vi "Square_Difference_Filter(SDisp)-2.vi"(5 "X,Y":dbl[][](array[numeric]), 6 "[IN] Dot matrix with \nstatuses for potentially \nmoving dots":i16[][](array[numeric]), 7 "Areas":dbl[][](array[numeric]), 8 "error IN":errorcluster, 9 "[IN] Possibly\nMoving (X,Y)":dbl[][](array[numeric]), 10 "% DIfference between \nParticle Squares":dbl, 11 "(X,Y,dX,dY) In":dbl[][](array[numeric])) -> (0 "error OUT":errorcluster, 1 "[OUT] Dot matrix with \nstatuses after searching \nof unmoving dots":i16[][](array[numeric]), 3 "[OUT] Filtered Single Displ (X,Y,dX,dY)":dbl[][](array[numeric]))   [LabVIEW 2013]
panel:
  out "Number \"+1\" events":i32
  out "Finded False Displac":i32
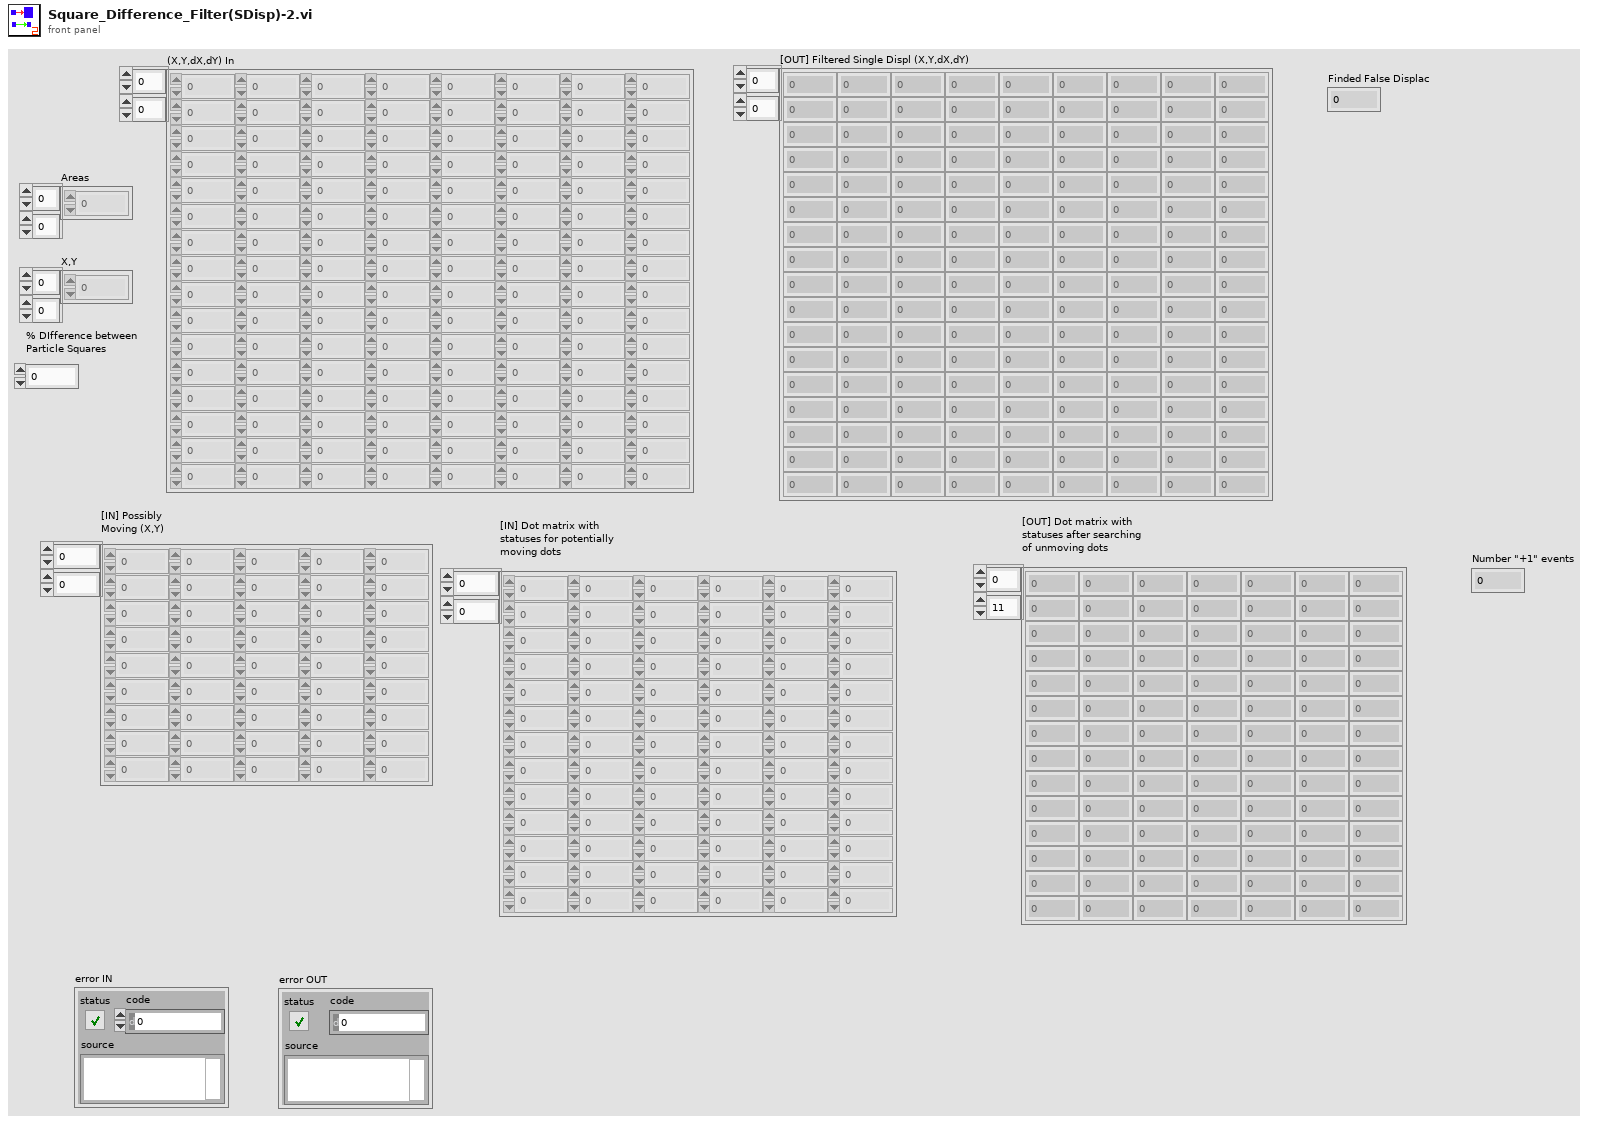
[diagram p1: front panel]
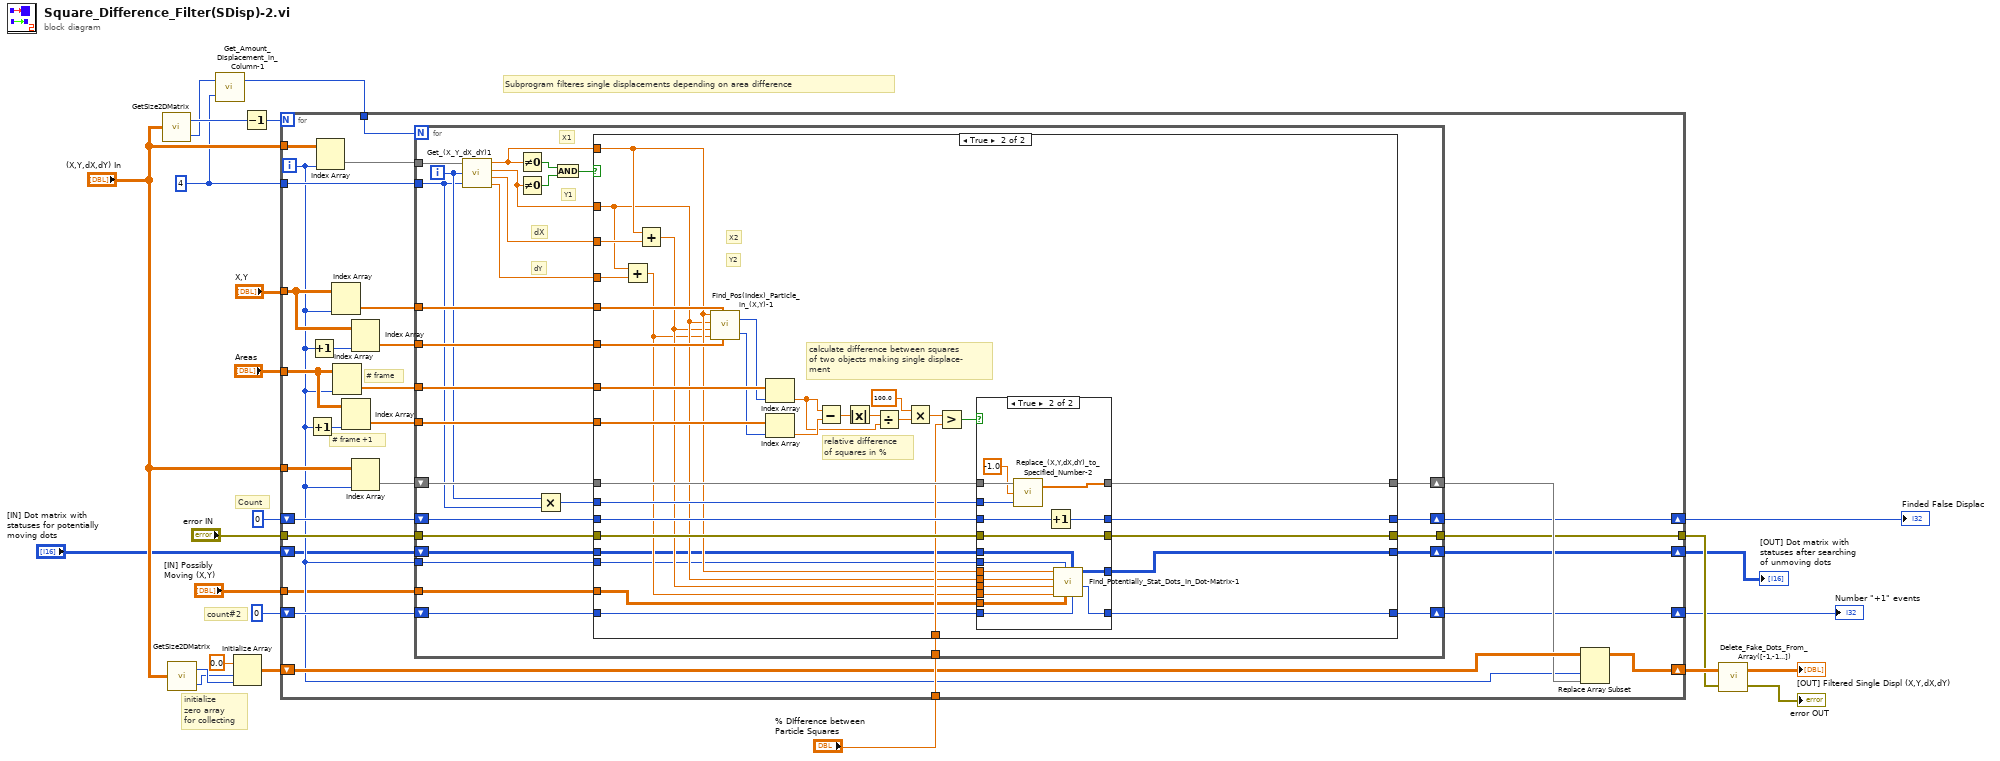
[diagram p0: block diagram]
diagram:
  w11 = 4 ("y")
  # "count#2"
  # "Subprogram filteres single displacements depending on area difference"
  # "initialize \nzero array \nfor collecting"
  # "Count"
  n1 = call "GetSize2DMatrix.vi"("Array IN (2D)"="(X,Y,dX,dY) In") -> ("# Cols"=w19:i32, "# Rows"=w12:i32)
  n2 = call "GetSize2DMatrix.vi"("Array IN (2D)"="(X,Y,dX,dY) In") -> ("# Cols"=w15:i32, "# Rows"=w14:i32)
  n3 = call "Get_Amount_Displacement_in_Column-1.vi"("multiplier"=w11, "# Rows"=w12) -> ("Displ amount"=w10:i32)  [unwired: 1 out]
  n4 = Initialize Array(0.0 ("element"), w14, w15) -> (w13:dbl[][])
  n5 = Decrement(x=w19) -> (x-1=w22:i32)
  n6 = for {
    N: w22 -> [_]
    tunnel: "error IN" -> [w53]
    tunnel: "(X,Y,dX,dY) In" -> [w52]
    shift-right: [w33] -> w23
    shift-left: 0 -> [w51]
    tunnel: "Areas" -> [w45]
    tunnel: "X,Y" -> [w50]
    tunnel: "% DIfference between \nParticle Squares" -> [w40]
    tunnel: "(X,Y,dX,dY) In" -> [w41]
    shift-right: [w37] -> w9
    shift-left: w13 -> [w38]
    tunnel: w11 -> [w36]
    tunnel: w10 -> [w35]
    shift-right: [w27] -> w2
    shift-left: 0 -> [w32]
    shift-right: [w28] -> w3
    shift-left: "[IN] Dot matrix with \nstatuses for potentially \nmoving dots" -> [w30]
    tunnel: "[IN] Possibly\nMoving (X,Y)" -> [w29]
    tunnel: [w26] -> w5
    i -> [w31]
    # "# frame"
    # "# frame +1"
    n7 = Increment(x=w31) -> (x+1=w46:i32)
    n8 = Increment(x=w31) -> (x+1=w49:i32)
    n9 = Index Array(array=w52, index (col)=w31) -> (element=w39:dbl[])  [unwired: 1 in]
    n10 = Index Array(array=w50, index (col)=w31) -> (element=w48:dbl[])  [unwired: 1 in]
    n11 = Index Array(array=w45, index (col)=w31) -> (element=w44:dbl[])  [unwired: 1 in]
    n12 = Index Array(array=w45, index (col)=w46) -> (element=w43:dbl[])  [unwired: 1 in]
    n13 = Index Array(array=w50, index (col)=w49) -> (element=w47:dbl[])  [unwired: 1 in]
    n14 = Index Array(array=w41, index (col)=w31) -> (element=w42:dbl[])  [unwired: 1 in]
    n15 = for {
      N: w35 -> [_]
      tunnel: w53 -> [w78]
      tunnel: w39 -> [w67]
      tunnel: [w77] -> w26
      shift-right: [w75] -> w33
      shift-left: w51 -> [w76]
      tunnel: w48 -> [w74]
      tunnel: w47 -> [w73]
      tunnel: w44 -> [w72]
      tunnel: w43 -> [w71]
      shift-right: [w69] -> w34
      shift-left: w42 -> [w70]
      tunnel: w40 -> [w68]
      tunnel: w36 -> [w61]
      shift-right: [w54] -> w27
      shift-left: w32 -> [w59]
      tunnel: w31 -> [w58]
      shift-right: [w56] -> w28
      shift-left: w30 -> [w57]
      tunnel: w29 -> [w55]
      i -> [w62]
      # "Y1"
      # "X1"
      # "dY"
      # "dX"
      n16 = call "Get_(X_Y_dX_dY)1.vi"("(X,Y,dX,dY)"=w67, "index"=w62, "multiplier"=w61) -> ("X"=w66:dbl, "Y"=w65:dbl, "dX"=w64:dbl, "dY"=w63:dbl)
      n17 = Not Equal To 0?(x=w66) -> (x != 0?=w81:bool)
      n18 = Not Equal To 0?(x=w65) -> (x != 0?=w80:bool)
      n19 = Multiply(x=w62, y=w61) -> (x*y=w60:i32)
      n20 = And(x=w81, y=w80) -> (x .and. y?=w79:bool)
      n21 = case shown="True" w79 {
        tunnel: w65 -> [_ w95]
        tunnel: w66 -> [_ w96]
        tunnel: w64 -> [_ w120]
        tunnel: w63 -> [_ w119]
        tunnel: [w86 w108] -> w77
        tunnel: w78 -> [w86 w107]
        tunnel: w76 -> [w85 w106]
        tunnel: [w85 w105] -> w75
        tunnel: w74 -> [_ w99]
        tunnel: w73 -> [_ w100]
        tunnel: w72 -> [_ w118]
        tunnel: w71 -> [_ w117]
        tunnel: w70 -> [w84 w104]
        tunnel: [w84 w103] -> w69
        tunnel: w68 -> [_ w102]
        tunnel: w60 -> [_ w101]
        tunnel: w59 -> [w82 w88]
        tunnel: w58 -> [_ w92]
        tunnel: w57 -> [w83 w91]
        tunnel: [w83 w90] -> w56
        tunnel: w55 -> [_ w89]
        tunnel: [w82 w87] -> w54
        frame False {
        }
        frame True {
          # "relative difference \nof squares in %"
          # "Y2"
          # "X2"
          # "calculate difference between squares\nof two objects making single displace-\nment"
          n22 = Add(x=w95, y=w119) -> (x+y=w93:dbl)
          n23 = Add(x=w96, y=w120) -> (x+y=w94:dbl)
          n24 = call "Find_Pos(Index)_Particle_in_(X,Y)-1.vi"("[X,Y] (n+1 Frame)"=w100, "[X,Y] (n Frame)"=w99, "Y2"=w93, "X2"=w94, "Y1"=w95, "X1"=w96) -> ("Index in (n+1) Frame"=w97:i32, "Index in (n) Frame"=w98:i32)
          n25 = Index Array(array=w118, index=w98) -> (element=w113:dbl)
          n26 = Index Array(array=w117, index=w97) -> (element=w116:dbl)
          n27 = Subtract(x=w113, y=w116) -> (x-y=w115:dbl)
          n28 = Absolute Value(x=w115) -> (abs(x)=w114:dbl)
          n29 = Divide(x=w114, y=w113) -> (x/y=w112:dbl)
          n30 = Multiply(x=100.0, y=w112) -> (x*y=w110:dbl)
          n31 = Greater?(x=w110, y=w102) -> (0:w109:bool)
          n32 = case shown="True" w109 {
            tunnel: [w123 w142] -> w108
            tunnel: w107 -> [w123 w142]
            tunnel: w106 -> [w125 w141]
            tunnel: [w125 w140] -> w105
            tunnel: w104 -> [w124 w139]
            tunnel: [w124 w126] -> w103
            tunnel: w101 -> [_ w138]
            tunnel: w96 -> [_ w136]
            tunnel: w95 -> [_ w135]
            tunnel: w94 -> [_ w134]
            tunnel: w93 -> [_ w133]
            tunnel: w92 -> [_ w132]
            tunnel: w91 -> [w122 w131]
            tunnel: [w122 w130] -> w90
            tunnel: w89 -> [_ w129]
            tunnel: w88 -> [w121 w128]
            tunnel: [w121 w127] -> w87
            frame False {
            }
            frame True {
              n33 = call "Replace_(X,Y,dX,dY)_to_Specified_Number-2.vi"("Starting index"=w138, "Replacement \nnumber"=-1.0 ("Replacement \nnumber"), "[IN] Sample \narray"=w139) -> ("[OUT] Processed\narray"=w126:dbl[])  [unwired: 1 out]
              n34 = Increment(x=w141) -> (x+1=w140:i32)
              n35 = call "Find_Potentially_Stat_Dots_In_Dot-Matrix-1.vi"("[IN] Count of event \"+1\""=w128, "[IN] Dot matrix with \nstatuses after searching \nof unmoving dots"=w131, "[IN] Possibly\nMoving (X,Y)"=w129, "Current # frame"=w132, "Y2"=w133, "X2"=w134, "Y1"=w135, "X1"=w136) -> ("[OUT] Count of event \"+1\" 2"=w127:i32, "[OUT] Dot matrix with \nstatuses after searching \nof unmoving dots"=w130:i16[][])  [unwired: 2 in]
            }
          }
        }
      }
    }
    n36 = Replace Array Subset(array=w38, new element=w34, index (col)=w31) -> (w37:dbl[][])  [unwired: 1 in]
  }
  "Finded False Displac" <- w23
  "[OUT] Dot matrix with \nstatuses after searching \nof unmoving dots" <- w3
  "Number \"+1\" events" <- w2
  n37 = call "Delete_Fake_Dots_From_Array([-1,-1...]).vi"("error IN"=w5, "Source Array"=w9) -> ("error OUT"=→"error OUT":errorcluster, "Filtered Array (X,Y,dX,dY)"=→"[OUT] Filtered Single Displ (X,Y,dX,dY)":dbl[][])
